vi "Switc CPP.vi"() -> ()   [LabVIEW 2017]
panel:
  out "String 3":string
  in  "Input SW type":u8(ring) items=["None", "Toggel ", "Moment. Up", "Moment. Down"]
  out "String 2":string
  in  "Serial baud":u8(ring)=9 items=["921600 bps"=1, "460800 bps"=2, "256000 bps"=3, "115200 bps"=4, "57600 bps"=5, "38400 bps"=6, "19200 bps"=7, "14400 bps"=8, "9600 bps"=9, "2400 bps"=10, "1200 bps"=11]
  in  "CAN baud":u8(ring)=4 items=["1000 kbps"=1, "800 kbps"=2, "500 kbps"=3, "250 kbps"=4, "125 kbps"=5, "100 kbps"=6, "83.3 kbps"=7, "62.5 kbps"=8, "50 kbps"=9, "20 kbps"=10, "10 kbps"=11]
  in  "Group control":u8(ring) items=["None", "Group 1 S", "Group 1 M", "Group 2 S", "Group 2 M", "Group 3 S", "Group 3 M", "Group 4 S", "Group 4 M", "Group 5 S", "Group 5 M", "Group 6 S", "Group 6 M"]
  out "String":string
  out "Strings []":string[](array[string])
  in  "Dig. Out control":u8(ring) items=["None", "OUT IN1", "OUT IN2", "OUT IN3", "OUT IN4", "Param. error", "Temp. error", "Voltage error", "spare", "BIT", "ANY CH status", "CH1 status", "CH2 status", "CH3 status", "CH4 status", "CH5 status", "CH6 status", "CH7 status", "CH8 status", "CH9 status", "CH10 status", "CH11 status", "CH12 status", "ANY CH. Trip", "CH1 Trip", "CH2 Trip", "CH3 Trip", "CH4 Trip", "CH5 Trip", "CH6 Trip", "CH7 Trip", "CH8 Trip", "CH9 Trip", "CH10 Trip", "CH11 Trip", "CH12 Trip", "ANY CH erorr"]
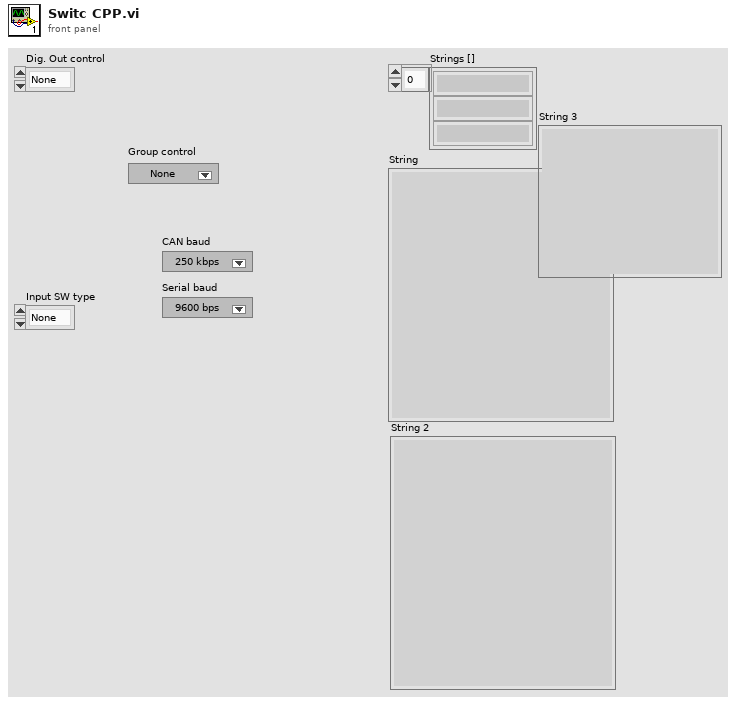
[diagram p1: front panel]
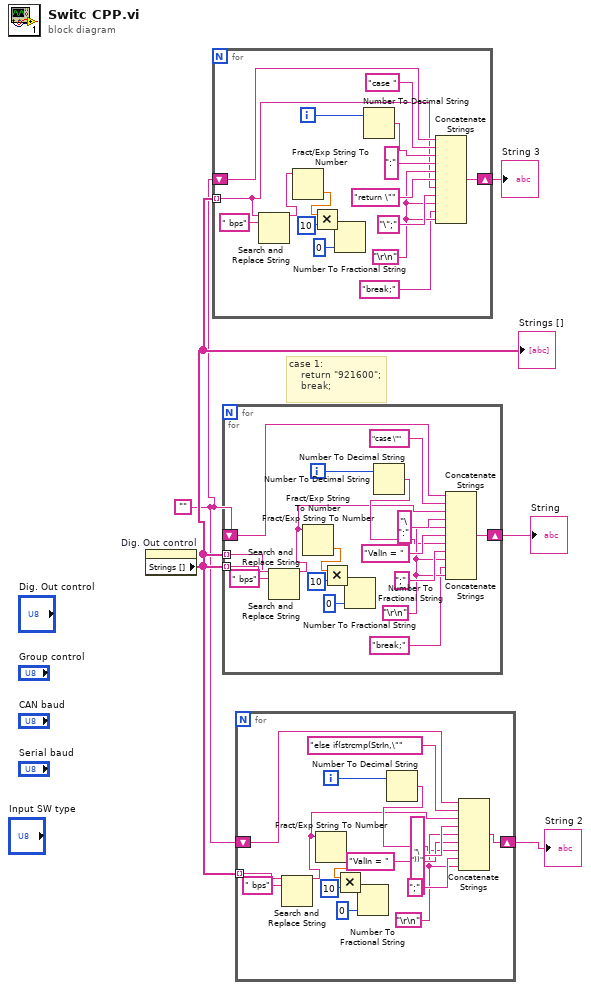
[diagram p0: block diagram]
diagram:
  w2 = ""
  # "case 1:\n\t\t\t\treturn \"921600\";\n\t\t\t\tbreak;"
  n1 = property on="Dig. Out control" class="Ring (strict)"() -> ("Strings []"=w3:string[])  [unwired: 2 in, 2 out]
  "Strings []" <- w3
  n2 = for {
    shift-right: [w16] -> w1
    shift-left: w2 -> [w15]
    tunnel: w3 -> [w6] mode=indexing
    i -> [w8]
    w18 = "\r\n"
    n3 = Search and Replace String(input string=w6, search string=" bps") -> (result string=w9:string)  [unwired: 6 in, 3 out]
    n4 = Fract/Exp String To Number(string=w9) -> (number=w10:dbl)  [unwired: 3 in, 1 out]
    n5 = Multiply(x=w10, y=10) -> (x*y=w13:dbl)
    n6 = Number To Fractional String(number=w13, precision (6)=i16 0) -> ()  [unwired: 2 in, 1 out]
    n7 = Number To Decimal String(number=w8) -> (decimal integer string=w7:string)  [unwired: 1 in]
    n8 = Concatenate Strings(w15, "case " ("string"), w7, ":" ("string"), w18, "return \"" ("string"), w6, "\";" ("string"), w18, "break;" ("string"), w18) -> (w16:string)
  }
  "String 3" <- w1
  n9 = for {
    shift-right: [w33] -> _
    shift-left: _ -> [w32]
    tunnel: w3 -> [w23] mode=indexing
    i -> [w24]
    w35 = "\r\n"
    n10 = Search and Replace String(input string=w23, search string=" bps") -> (result string=w25:string)  [unwired: 6 in, 3 out]
    n11 = Fract/Exp String To Number(string=w25) -> (number=w26:dbl)  [unwired: 3 in, 1 out]
    n12 = Multiply(x=w26, y=10) -> (x*y=w29:dbl)
    n13 = Number To Fractional String(number=w29, precision (6)=i16 0) -> ()  [unwired: 2 in, 1 out]
    n14 = Number To Decimal String(number=w24) -> (decimal integer string=w31:string)  [unwired: 1 in]
    n15 = Concatenate Strings(w32, "case \"" ("string"), w25, "\":" ("string"), w35, "ValIn = " ("string"), w31, ";" ("string"), w35, "break;" ("string"), w35) -> (w33:string)
  }
  n16 = for {
    tunnel: w3 -> [w42] mode=indexing
    shift-right: [w50] -> w5
    shift-left: w2 -> [w49]
    i -> [w40]
    w52 = "\r\n"
    n17 = Search and Replace String(input string=w42, search string=" bps") -> (result string=w41:string)  [unwired: 6 in, 3 out]
    n18 = Fract/Exp String To Number(string=w41) -> (number=w43:dbl)  [unwired: 3 in, 1 out]
    n19 = Multiply(x=w43, y=10) -> (x*y=w46:dbl)
    n20 = Number To Fractional String(number=w46, precision (6)=i16 0) -> ()  [unwired: 2 in, 1 out]
    n21 = Number To Decimal String(number=w40) -> (decimal integer string=w48:string)  [unwired: 1 in]
    n22 = Concatenate Strings(w49, "case \"" ("string"), w41, "\":" ("string"), w52, "ValIn = " ("string"), w48, ";" ("string"), w52, "break;" ("string"), w52) -> (w50:string)
  }
  "String" <- w5
  n23 = for {
    tunnel: w3 -> [w59] mode=indexing
    shift-right: [w67] -> w4
    shift-left: w2 -> [w66]
    i -> [w57]
    w68 = "\r\n"
    n24 = Search and Replace String(input string=w59, search string=" bps") -> (result string=w58:string)  [unwired: 6 in, 3 out]
    n25 = Fract/Exp String To Number(string=w58) -> (number=w60:dbl)  [unwired: 3 in, 1 out]
    n26 = Multiply(x=w60, y=10) -> (x*y=w63:dbl)
    n27 = Number To Fractional String(number=w63, precision (6)=i16 0) -> ()  [unwired: 2 in, 1 out]
    n28 = Number To Decimal String(number=w57) -> (decimal integer string=w65:string)  [unwired: 1 in]
    n29 = Concatenate Strings(w66, "else if(strcmp(StrIn,\"" ("string"), w58, "\"))" ("string"), w68, "ValIn = " ("string"), w65, ";" ("string"), w68) -> (w67:string)
  }
  "String 2" <- w4
